vi "getSpectrumFromFile.vi"(10 "end of header":string="f.E(f)\n", 11 "File Path Control":path) -> (2 "array":dbl[][](array[numeric]))   [LabVIEW 2013]
panel:
  out "The Data":string
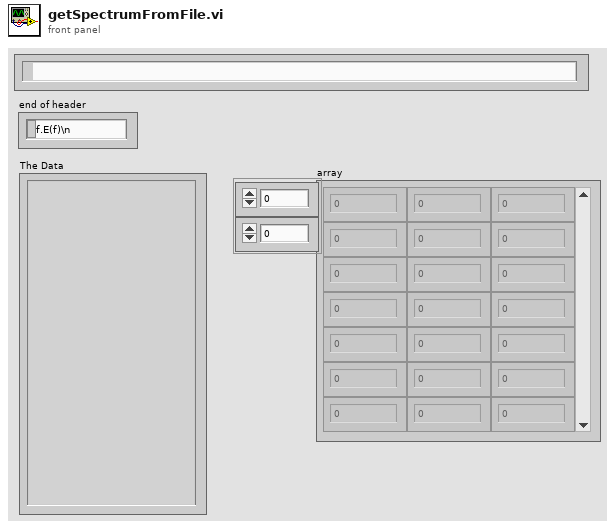
[diagram p1: front panel]
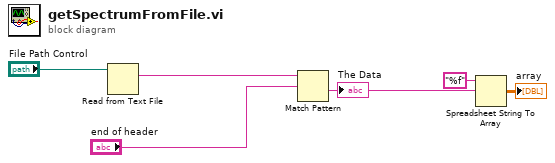
[diagram p0: block diagram]
diagram:
  n1 = Read from Text File(file (use dialog)="File Path Control") -> (text=w4:string)  [unwired: 3 in, 3 out]
  n2 = Match Pattern(string=w4, regular expression="end of header") -> (after substring=w3:string)  [unwired: 1 in, 3 out]
  "The Data" <- w3
  n3 = Spreadsheet String To Array(format string="%f", spreadsheet string=w3) -> (array=→"array":dbl[][])  [unwired: 2 in]
